vi "VCS Open SubDevice.vi"(8 "error in (no error)":errorcluster, 10 "deviceHandle":u32, 11 "device in":T1={"deviceName"="EPOS2", "protocolStackName"="CANopen"}) -> (0 "error out":errorcluster, 3 "keyHandle out":u32)   [LabVIEW 2019, in "maxonEPOS.lvlib"]
doc: "<B>VCS Open SubDevice</B> opens the subdevice connected to gateway device to send and receive commands."
uses:
  Examples/maxonEPOS.lvlib
  Resources/EposCmd.dll
  Resources/EposCmd64.dll
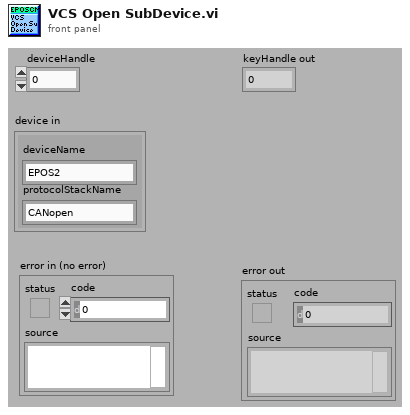
[diagram p1: front panel]
types:
  T1 = cluster{"deviceName":string, "protocolStackName":string}
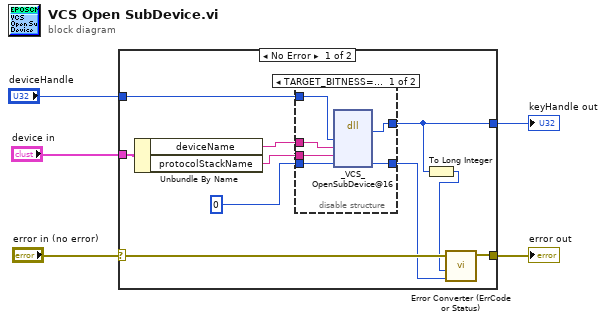
[diagram p0: block diagram]
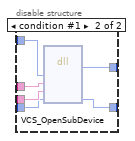
[diagram p2: hidden frame]
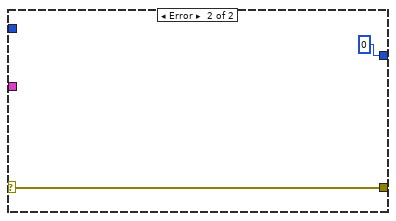
[diagram p3: hidden frame]
diagram:
  n1 = case shown="No Error" "error in (no error)" {
    selector: "error in (no error)" -> [w15 w29]
    tunnel: [w14 w29] -> w4
    tunnel: "device in" -> [w12 _]
    tunnel: [w6 u32 0] -> w2
    tunnel: "deviceHandle" -> [w8 _]
    frame No Error {
      n2 = Unbundle By Name(w12) -> ("deviceName"=w11:string, "protocolStackName"=w10:string)
      n3 = disable-structure shown="TARGET_BITNESS==32, Standard" {
        disable-tunnel: [w21 w27] -> w13
        disable-tunnel: w11 -> [w20 w26]
        disable-tunnel: w10 -> [w19 w25]
        disable-tunnel: u32 0 ("pErrorCode") -> [w18 w24]
        disable-tunnel: [w17 w23] -> w6
        disable-tunnel: w8 -> [w16 w22]
        frame condition #0 (active) {
          n4 = dll-call lib="C:/workspace/project/scancon/sw/SSI_Tool/InstrumentsInterfaces/Motordriver/maxon EPOS/Resources/EposCmd.dll" fn="_VCS_OpenSubDevice@16"("deviceHandle"=w16, "DeviceName"=w20, "ProtocolStackName"=w19, "pErrorCode"=w18) -> ("Rückgabetyp"=w17:u32, "pErrorCode"=w21:u32)  [unwired: 6 in, 2 out]
        }
        frame condition #1 {
          n5 = dll-call lib="C:/Sources/LabView/maxon EPOS/Resources/EposCmd64.dll" fn="VCS_OpenSubDevice"("deviceHandle"=w22, "DeviceName"=w26, "ProtocolStackName"=w25, "pErrorCode"=w24) -> ("return type"=w23:u32, "pErrorCode"=w27:u32)  [unwired: 6 in, 2 out]
        }
      }
      n6 = To Long Integer(number=w6) -> (32bit integer=w7:i32)
      n7 = call "Error Converter (ErrCode or Status).vi"("error code"=w13, "return type"=w7, "error in (no error)"=w15) -> ("error out"=w14:errorcluster)  [unwired: 7 in]
    }
    frame Error {
    }
  }
  "error out" <- w4
  "keyHandle out" <- w2
